vi "Mapped Pixel Pointer Example.vi"() -> ()   [LabVIEW 2020, in "examples.lvlib"]
doc: "Demonstrate the Mapped Pixel Pointer Example which provides access to the underlying memory of an Image. This can be used with other Toolkits and Libraries that operate on pointers to memory."
uses:
  examples.lvlib
  image/ARGB Colour.ctl
  common/Image Size (Integer).ctl
  image/Mapped Memory Access Image ARGB/Mapped Memory Access Image ARGB.lvclass/Mapped Memory Access Image ARGB.ctl
  image/New Image (ARGB Preallocated).vi
  image/Mapped Memory Access Image ARGB/Acquire.vi
  image/Mapped Memory Access Image ARGB/Get Mapped Memory Infomation.vi
  image/Mapped Memory Access Image ARGB/Release.vi
  image/Draw Image to Picture (ARGB).vi
  image/New Image (ARGB Preallocated).vi/3321fa97-f432-4e1e-8db9-a0df79aed21b.vi
  image/ARGB Colour to U32 Pixel Value.vi
  image/Draw Image to Picture (ARGB).vi/8cd07b1b-062e-4fe4-9e87-2eb3dc89fe0e.vi
  <vilib>/Utility/error.llb/Error Cluster From Error Code.vi
  image/Mapped Memory Access Image ARGB/Mapped Memory Access Image ARGB.lvclass
  image/image.lvlib
  common/common.lvlib
panel:
  out "Picture":picture
  out "Starting Data":u32[][](array[numeric])
  out "Output Data":u32[][](array[numeric])
  out "error out":errorcluster
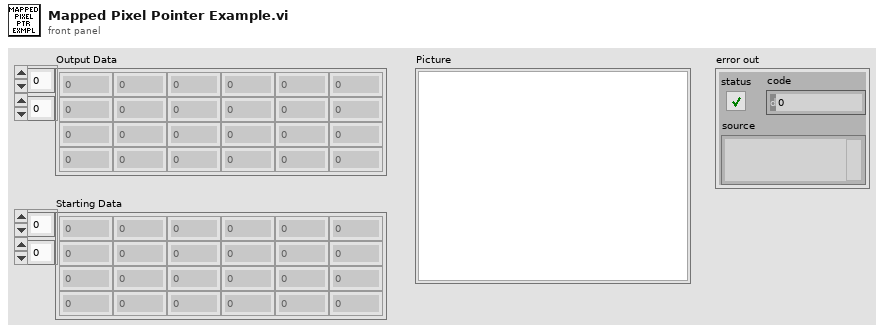
[diagram p1: front panel]
types:
  T1 = typedef "common.lvlib/Image Size (Integer).ctl" = cluster{"Width":u16, "Height":u16}
  T2 = typedef "image.lvlib/ARGB Colour.ctl" = cluster{"Alpha":u8, "RGB":u32}
  T3 = typedef "image.lvlib/ARGB Image.ctl" = refnum<data-value>
  T4 = typedef "image.lvlib/Raw Memory Information.ctl" = cluster{"Memory Address":u64, "Dimension 0":T5, "Dimension 1":T5}
  T5 = typedef "image.lvlib/Raw Memory Information Dimension.ctl" = cluster{"Size":u16, "Stride":i32}
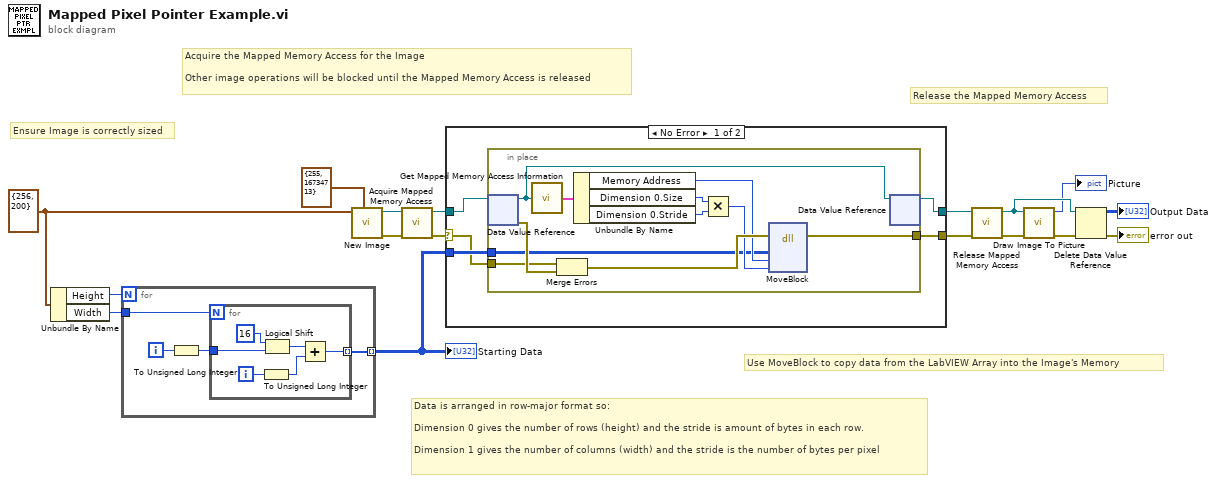
[diagram p0: block diagram]
diagram:
  w13 = T1 {"Width"=256, "Height"=200} ("Preallocated Image Size (Default: 0,0)")
  # "Release the Mapped Memory Access"
  # "Ensure Image is correctly sized"
  # "Use MoveBlock to copy data from the LabVIEW Array into the Image's Memory"
  # "Data is arranged in row-major format so: \n\nDimension 0 gives the number of rows (height) and the stride is amount of bytes in each row. \n\nDimension 1 gives the number of columns (width) and the stride is the number of bytes per pixel"
  # "Acquire the Mapped Memory Access for the Image\n\nOther image operations will be blocked until the Mapped Memory Access is released"
  n1 = Unbundle By Name(w13) -> ("Height"=w10:u16, "Width"=w12:u16)
  n2 = for {
    N: w10 -> [_]
    tunnel: w12 -> [w21]
    tunnel: [w18] -> w11 mode=indexing
    i -> [w20]
    n3 = To Unsigned Long Integer(number=w20) -> (unsigned 32bit integer=w19:u32)
    n4 = for {
      N: w21 -> [_]
      tunnel: w19 -> [w26]
      tunnel: [w22] -> w18 mode=indexing
      i -> [w27]
      n5 = To Unsigned Long Integer(number=w27) -> (unsigned 32bit integer=w23:u32)
      n6 = Logical Shift(y=i16 16, x=w26) -> (x << y=w25:u32)
      n7 = Add(x=w25, y=w23) -> (x+y=w22:u32)
    }
  }
  "Starting Data" <- w11
  n8 = call-poly "New Image.vi"("Colour (Default: Black)"=T2 {"Alpha"=255, "RGB"=16734713}, "Preallocated Image Size (Default: 0,0)"=w13) -> ("error out"=w16:errorcluster, "ARGB Image"=w8:T3)  [unwired: 8 in]
  n9 = call-poly "Acquire Mapped Memory Access.vi"("error in (no error)"=w16, "Image in"=w8) -> ("error out"=w7:errorcluster, "Mapped Memory Access Image ARGB"=w15:refnum<data-value>)  [unwired: 8 in]
  n10 = case shown="No Error" w7 {
    selector: w7 -> [w29 w44]
    tunnel: w15 -> [w32 w45]
    tunnel: [w31 w45] -> w14
    tunnel: w11 -> [w30 _]
    tunnel: [w28 w44] -> w6
    frame No Error {
      n11 = in-place {
        in-place-border: w30 -> [w33]
        in-place-border: w29 -> [w35]
        in-place-border: [w34] -> w28
        n12 = in-place-dvr #1(w32) -> (w42:refnum<class "Mapped Memory Access Image ARGB.lvclass">, w36:errorcluster)
        n13 = call-poly "Get Mapped Memory Access Information.vi"("Mapped Memory Access Image ARGB in"=w42) -> ("Raw Memory Information"=w41:T4)
        n14 = Merge Errors(w35, w36) -> (w43:errorcluster)
        n15 = Unbundle By Name(w41) -> ("Memory Address"=w40:u64, "Dimension 0.Size"=w39:u16, "Dimension 0.Stride"=w38:i32)
        n16 = Multiply(x=w39, y=w38) -> (x*y=w37:i32)
        n17 = dll-call lib="LabVIEW" fn="MoveBlock"(error in=w43, "source"=w33, "destination"=w40, "size"=w37) -> (error out=w34:errorcluster)  [unwired: 6 in, 1 out]
        n18 = in-place-dvr #1(w42) -> (w31:refnum<data-value>)  [unwired: 1 out]
      }
    }
    frame Error {
    }
  }
  n19 = call-poly "Release Mapped Memory Access.vi"("error in (no error)"=w6, "Mapped Memory Access Image ARGB"=w14) -> ("error out"=w3:errorcluster, "Image ARGB"=w4:T3)  [unwired: 8 in]
  n20 = call-poly "Draw Image To Picture.vi"("error in (no error)"=w3, "ARGB Image Source in"=w4) -> ("error out"=w2:errorcluster, "Picture"=→"Picture":picture)  [unwired: 8 in]
  n21 = Delete Data Value Reference(data value reference=w4, error in=w2) -> (data value=→"Output Data":u32[][], error out=→"error out":errorcluster)
